vi "Temp_Splitter_SUBVI.vi"(10 "DAQ_OUT":dbl[](array[numeric]), 11 "Tomt Array":dbl[](array[numeric])) -> (0 "Counter_Array":dbl[](array[numeric]), 1 "TEMP3":dbl[](array[numeric]), 2 "TEMP2":dbl[](array[numeric]), 3 "TEMP1":dbl[](array[numeric]))   [LabVIEW 2022 SP3]
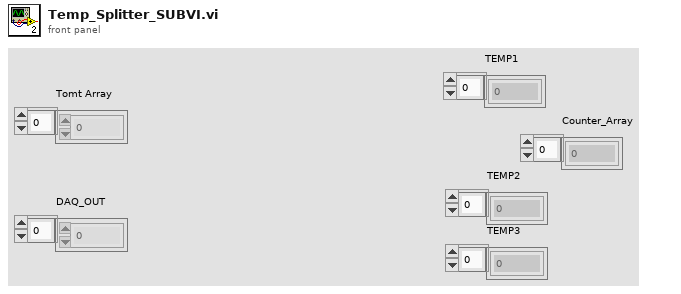
[diagram p1: front panel]
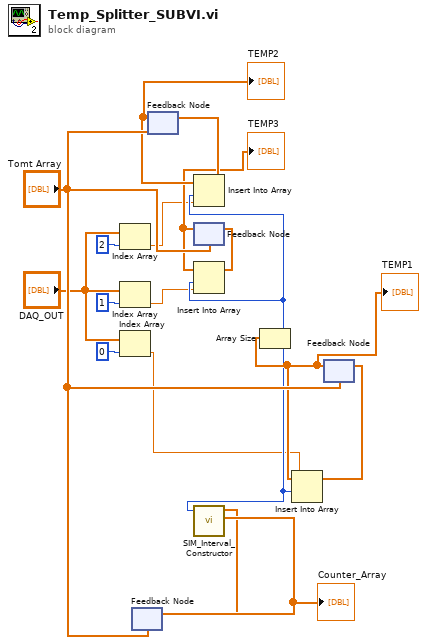
[diagram p0: block diagram]
diagram:
  n1 = Index Array(array="DAQ_OUT", index=2) -> (element=w5:dbl)
  n2 = Index Array(array="DAQ_OUT", index=1) -> (element=w6:dbl)
  n3 = Index Array(array="DAQ_OUT", index=0) -> (element=w4:dbl)
  n4 = feedback #1("Tomt Array") -> (w17:dbl[])
  "Counter_Array" <- w17
  n5 = feedback #2("Tomt Array") -> (w14:dbl[])
  "TEMP2" <- w14
  n6 = feedback #3("Tomt Array") -> (w12:dbl[])
  "TEMP3" <- w12
  n7 = feedback #4("Tomt Array") -> (w10:dbl[])
  "TEMP1" <- w10
  n8 = Array Size(array=w10) -> (size(s)=w8:i32)
  n9 = Insert Into Array(array=w14, index=w8, new element=w5) -> (w13:dbl[])
  n10 = feedback-in #2(w13) -> ()
  n11 = Insert Into Array(array=w12, index=w8, new element=w6) -> (w11:dbl[])
  n12 = feedback-in #3(w11) -> ()
  n13 = call "SIM_Interval_Constructor.vi"("History Data in"=w17, "size(s)"=w8) -> ("History Data out"=w16:dbl[])  [unwired: 9 in]
  n14 = feedback-in #1(w16) -> ()
  n15 = Insert Into Array(array=w10, index=w8, new element=w4) -> (w9:dbl[])
  n16 = feedback-in #4(w9) -> ()
